vi "_SetIsNapping.vi"(8 "error in (no error)":errorcluster, 10 "IsNapping (F)":bool, 11 "Baby in":refnum<class "Baby.lvclass">) -> (0 "error out":errorcluster, 3 "Baby out":refnum<class "Baby.lvclass">)   [LabVIEW 2009, in "Baby.lvclass"]
uses:
  Baby.lvclass
  Baby.lvclass/Baby.ctl
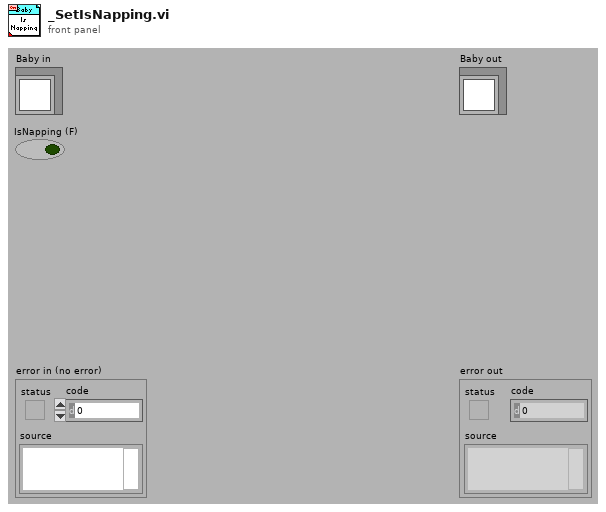
[diagram p1: front panel]
types:
  T1 = typedef "Baby.lvclass/_PrivateDataDvr.ctl" = refnum<data-value>
  T2 = typedef "Baby.lvclass/_PrivateData.ctl" = cluster{"IsNapping":bool}
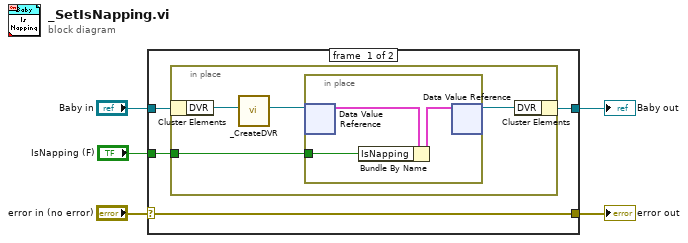
[diagram p0: block diagram]
diagram:
  n1 = case shown="No Error" "error in (no error)" {
    selector: "error in (no error)" -> [w9 w18]
    tunnel: [w9 w18] -> w4
    tunnel: [w7 w17] -> w2
    tunnel: "Baby in" -> [w8 w17]
    tunnel: "IsNapping (F)" -> [w6 _]
    frame #0 {
      n2 = in-place {
        in-place-border: w6 -> [w12]
        n3 = in-place-cluster #1(w8) -> ("DVR"=w11:T1)
        n4 = call "_CreateDVR.vi"("PrivateDataDvr"=w11) -> ("PrivateDataDvr out"=w10:T1)  [unwired: 10 in]
        n5 = in-place {
          in-place-border: w12 -> [w14]
          n6 = in-place-dvr #2(w10) -> (w16:T2)  [unwired: 1 out]
          n7 = Bundle By Name(cluster=w16, "IsNapping"=w14) -> (w15:T2)
          n8 = in-place-dvr #2(w15) -> (w13:T1)  [unwired: 1 out]
        }
        n9 = in-place-cluster #1("DVR"=w13) -> (w7:refnum<class "Baby.lvclass">)
      }
    }
    frame #1 {
    }
  }
  "error out" <- w4
  "Baby out" <- w2
